vi "TCP-IP Mgr.Get Config.vi"(8 "error in":errorcluster, 10 "Default Config":T1={"IP"="127.0.0.1", "Port"=8500, "Dir"=FALSE}, 11 "Path":path=path "C:/TestExec/Config/TESocket.ini") -> (0 "error out":errorcluster, 2 "Config Out":T1={"IP"="127.0.0.1", "Port"=8500, "Dir"=FALSE})   [LabVIEW 2017, in "TCP-IP Mgr.lvlib"]
uses:
  TCP-IP Mgr.lvlib
  TCP-IP Mgr.Config.ctl
  <vilib>/Utility/config.llb/Read Key (String).vi
  <vilib>/Utility/config.llb/Write Key (String).vi
  <vilib>/Utility/config.llb/Read Key (I32).vi
  <vilib>/Utility/config.llb/Write Key (I32).vi
  <vilib>/Utility/config.llb/NI_LVConfig.lvlib
  <vilib>/KATE/Files/File Utils.lvlib
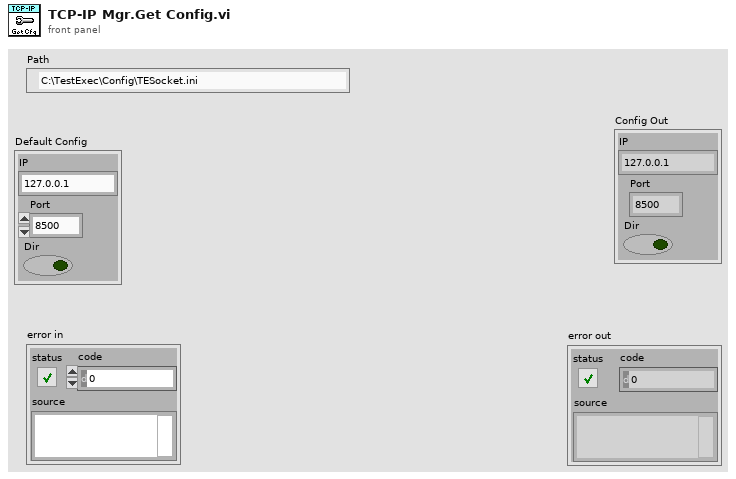
[diagram p1: front panel]
types:
  T1 = typedef "TCP-IP Mgr.lvlib/TCP-IP Mgr.Config.ctl" = cluster{"IP":string, "Port":u16, "Dir":bool}
  T2 = typedef "NI_LVConfig.lvlib/Config Data RefNum.ctl" = refnum<k1>
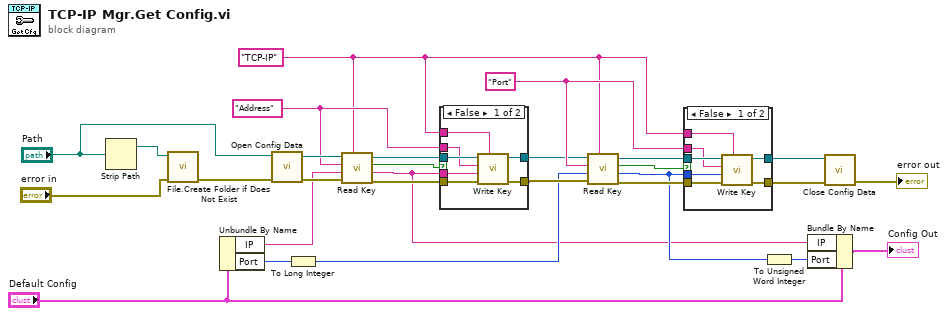
[diagram p0: block diagram]
diagram:
  w16 = "Port"
  w21 = "Address"
  w14 = "TCP-IP"
  n1 = Strip Path(path="Path") -> (stripped path=w4:path)  [unwired: 1 out]
  n2 = call <vilib>:"File.Create Folder if Does Not Exist.vi"("error in"="error in", "Path"=w4) -> ("error out"=w2:errorcluster)  [unwired: 7 in, 2 out]
  n3 = Unbundle By Name("Default Config") -> ("IP"=w26:string, "Port"=w24:u16)
  n4 = call <vilib>:"Open Config Data.vi"("error in (no error)"=w2, "configuration file path"="Path") -> ("error out"=w28:errorcluster, "refnum"=w27:T2)  [unwired: 7 in, 1 out]
  n5 = To Long Integer(number=w24) -> (32bit integer=w11:i32)
  n6 = call-poly <vilib>:"Read Key.vi"("section"=w14, "error in (no error)"=w28, "default value"=w26, "key"=w21, "refnum"=w27) -> ("error out"=w22:errorcluster, "value"=w9:string, "found?"=w19:bool, "refnum out"=w20:T2)  [unwired: 3 in]
  n7 = case shown="False" w19 {
    tunnel: w22 -> [w35 w36]
    tunnel: w9 -> [w34 _]
    tunnel: w21 -> [w32 _]
    tunnel: w20 -> [w33 w37]
    tunnel: w14 -> [w31 _]
    tunnel: [w30 w37] -> w13
    tunnel: [w29 w36] -> w12
    frame False {
      n8 = call-poly <vilib>:"Write Key.vi"("section"=w31, "error in (no error)"=w35, "value"=w34, "key"=w32, "refnum"=w33) -> ("error out"=w29:errorcluster, "refnum out"=w30:T2)  [unwired: 4 in, 1 out]
    }
    frame True {
    }
  }
  n9 = call-poly <vilib>:"Read Key.vi"("section"=w14, "error in (no error)"=w12, "default value"=w11, "key"=w16, "refnum"=w13) -> ("error out"=w15:errorcluster, "value"=w10:i32, "found?"=w18:bool, "refnum out"=w17:T2)  [unwired: 3 in]
  n10 = case shown="False" w18 {
    tunnel: w15 -> [w44 w45]
    tunnel: w10 -> [w43 _]
    tunnel: w16 -> [w41 _]
    tunnel: w17 -> [w42 w46]
    tunnel: w14 -> [w40 _]
    tunnel: [w39 w46] -> w8
    tunnel: [w38 w45] -> w7
    frame False {
      n11 = call-poly <vilib>:"Write Key.vi"("section"=w40, "error in (no error)"=w44, "value"=w43, "key"=w41, "refnum"=w42) -> ("error out"=w38:errorcluster, "refnum out"=w39:T2)  [unwired: 4 in, 1 out]
    }
    frame True {
    }
  }
  n12 = To Unsigned Word Integer(number=w10) -> (unsigned 16bit integer=w25:u16)
  n13 = Bundle By Name(cluster="Default Config", "IP"=w9, "Port"=w25) -> (→"Config Out":T1)
  n14 = call <vilib>:"Close Config Data.vi"("error in (no error)"=w7, "refnum"=w8) -> ("error out"=→"error out":errorcluster)  [unwired: 8 in, 1 out]
